vi "Set_Hi-Tec_server.vi"(4 "Client Name":string, 6 "Density Ratio":string, 7 "Strength (% by volume)":dbl min=0.0 max=5.0 format="%.3f", 8 "Stack flowrate (l/min)":dbl format="%.2f", 9 "Mode":enum16{"Control Hi-Tec", "Check Hi-Tec Demands"}(ring)) -> (0 "Flowrates (kg/min)":dbl[](array[numeric]) format="%.2f", 1 "Comment":string)   [LabVIEW 2014]
uses:
  ADAM Client/Sub VIs/ADAM Controls/Ch_description_ADAM.ctl
  ADAM Client/Sub VIs/ADAM Controls/Module_type_ADAM.ctl
  ADAM Client/Sub VIs/ADAM Controls/Function_ADAM.ctl
  ADAM Client/Sub VIs/ADAM Controls/Channel_State.ctl
  ADAM Client/Sub VIs/ADAM Controls/Calib_type_ADAM.ctl
  ADAM Client/Sub VIs/ADAM Controls/Address.ctl
  ADAM Client/Sub VIs/ADAM Controls/Update_scan_value.ctl
  Anemometry/Anemometry Sub Vis/Globals/Gas_management_global.vi
panel:
  # "-Carrier 1 only\n-Carrier 2 only\n-Enter Ratio"
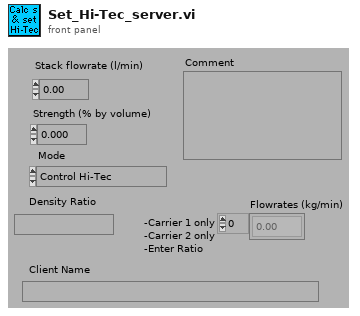
[diagram p1: front panel]
types:
  T1 = enum16{"Append to Global", "Read Global then Clear"}
  T2 = typedef "Calib_type_ADAM.ctl" = enum16{"Raw", "Bx + A", "Cx^2 + Bx + A", "Dx^3 + Cx^2 + Bx + A", "In Band", "Hi-Tec Q", "Hi-Tec M_dot", "Text"}
  T3 = typedef "Module_type_ADAM.ctl" = string
  T4 = typedef "Ch_description_ADAM.ctl" = cluster{"Ch Name":string, "Type":T3, "Function":T5, "Ch State":T6, "Calibration type":T2, "A":dbl, "B":dbl, "C":dbl, "D":dbl, "Comments":string, "Address":T7, "String":string, "Duty":u16}
  T5 = typedef "Function_ADAM.ctl" = enum16{"Analogue Input", "Digital Input", "Event counter", "Event rate", "Analogue Output", "Digital Output", "Relay Output"}
  T6 = typedef "Channel_State.ctl" = enum16{"On", "Off", "Always On", "Always Off"}
  T7 = typedef "Address.ctl" = cluster{"Main":i32, "Ch.":i32, "Sub":i32, "Port Name":string}
  T8 = typedef "Update_scan_value.ctl" = cluster{"Channel Name":string, "New Value":dbl}
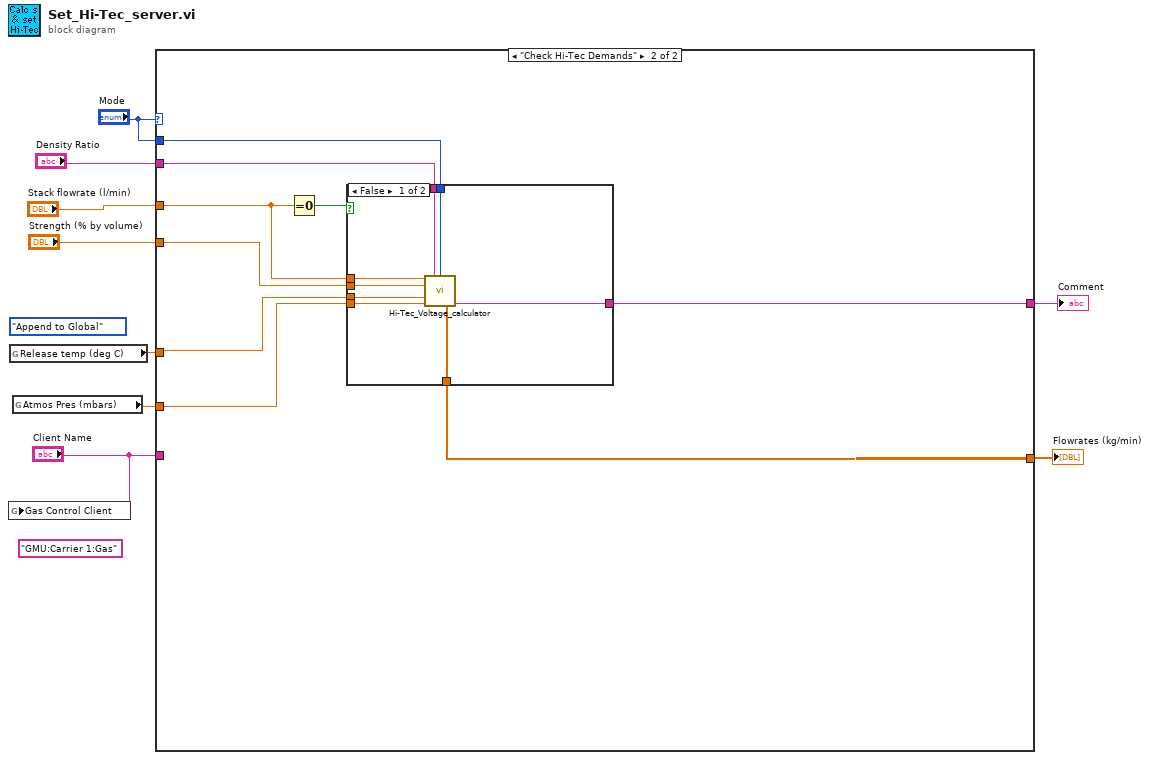
[diagram p0: block diagram]
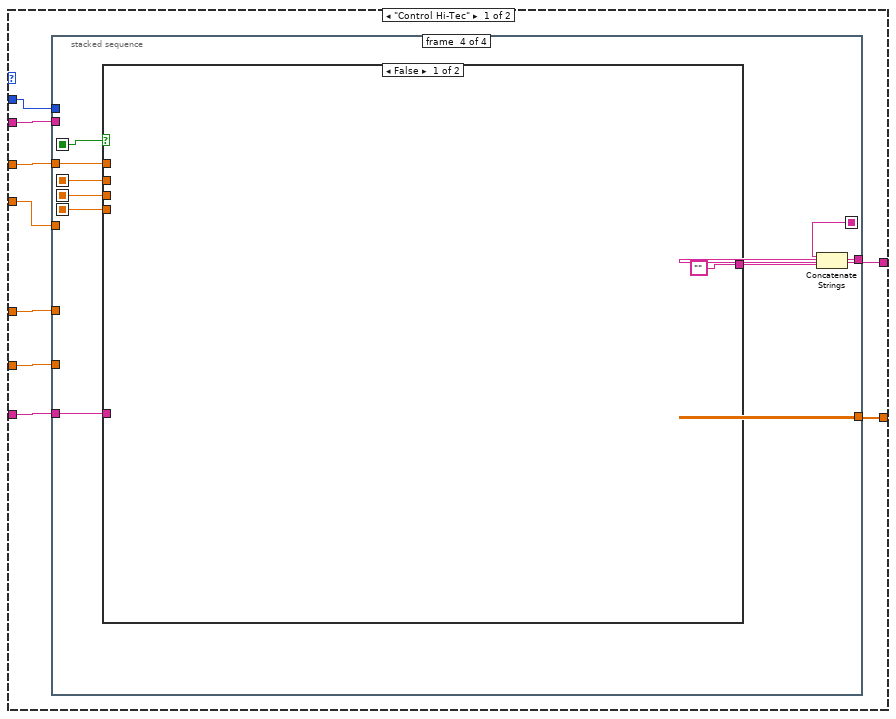
[diagram p2: hidden frame]
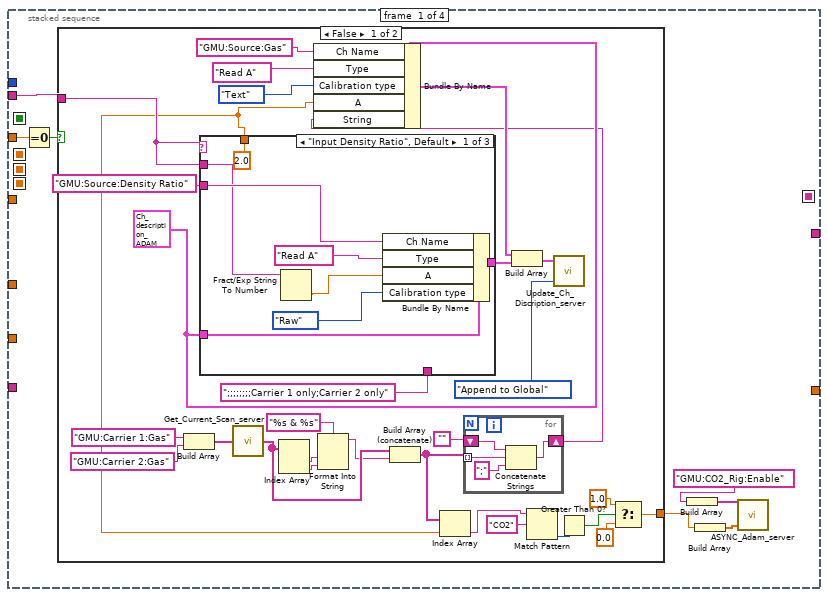
[diagram p3: hidden frame]
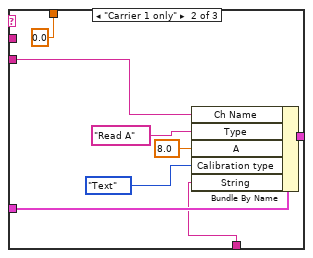
[diagram p4: hidden frame]
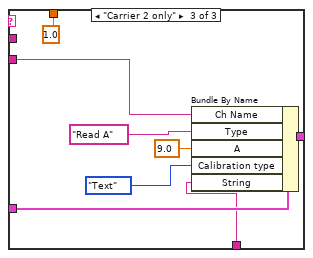
[diagram p5: hidden frame]
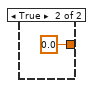
[diagram p6: hidden frame]
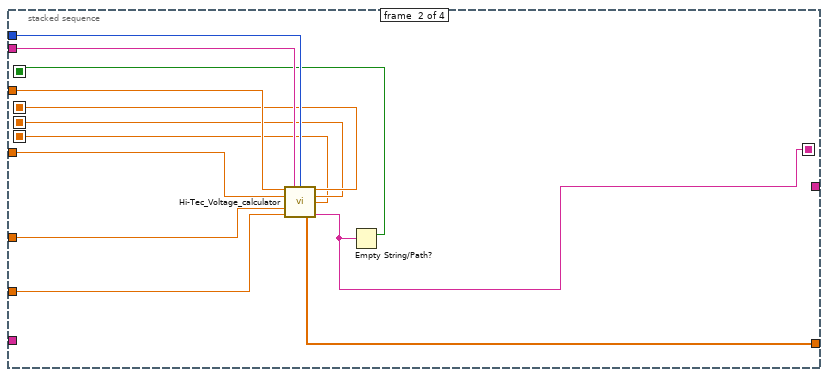
[diagram p7: hidden frame]
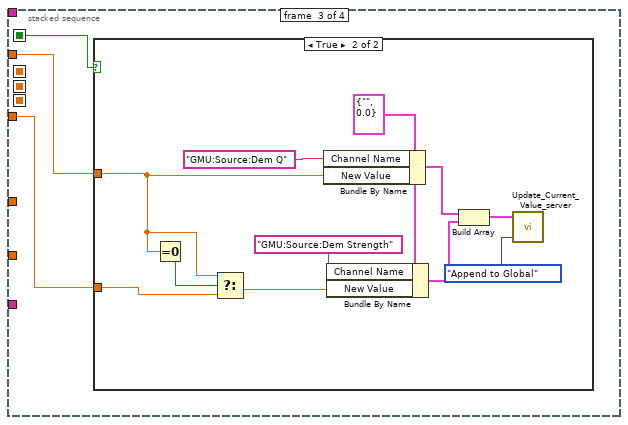
[diagram p8: hidden frame]
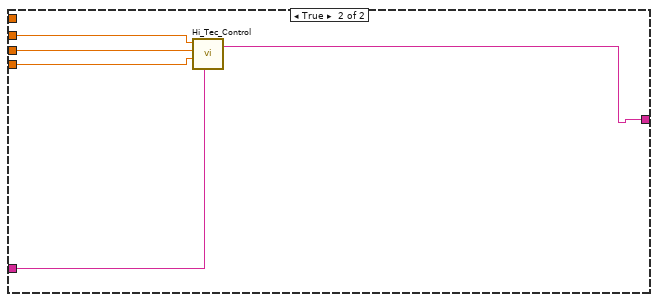
[diagram p10: hidden frame]
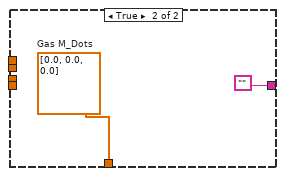
[diagram p11: hidden frame]
diagram:
  (unwired) T1."Append to Global" ("Mode")
  (unwired) "GMU:Carrier 1:Gas"
  n1 = global write "Gas_management_global.vi" "Gas Control Client"("Client Name") -> ()
  n2 = global read "Gas_management_global.vi" "Release temp (deg C)"() -> (w5:dbl)
  n3 = global read "Gas_management_global.vi" "Atmos Pres (mbars)"() -> (w7:dbl)
  n4 = case shown="\"Check Hi-Tec Demands\"" "Mode" {
    tunnel: "Density Ratio" -> [w18 w131]
    tunnel: "Strength (% by volume)" -> [w17 w134]
    tunnel: "Stack flowrate (l/min)" -> [w16 w129]
    tunnel: w5 -> [w15 w133]
    tunnel: w7 -> [w14 w132]
    tunnel: [w13 w130] -> w6
    tunnel: [w12 w127] -> w3
    tunnel: "Mode" -> [w11 w126]
    tunnel: "Client Name" -> [w10 _]
    frame "Control Hi-Tec" {
      n5 = stacked-sequence {
        seq-local: [_ w89 _ _] -> [_ _ w97 w115]
        seq-local: [_ w88 _ _] -> [_ _ _ w119]
        seq-local: [_ w87 _ _] -> [_ _ _ w118]
        seq-local: [_ w86 _ _] -> [_ _ _ w117]
        seq-local: [_ w85 _ _] -> [_ _ _ w112]
        tunnel: w18 -> [w25 w94 _ _]
        tunnel: w17 -> [_ w93 w98 _]
        tunnel: w16 -> [w24 w92 w99 w114]
        tunnel: w15 -> [_ w96 _ _]
        tunnel: w14 -> [_ w95 _ _]
        tunnel: [_ _ _ w113] -> w13
        tunnel: [_ w91 _ _] -> w12
        tunnel: w11 -> [_ w90 _ _]
        tunnel: w10 -> [_ _ _ w116]
        frame #0 {
          n6 = Equal To 0?(x=w24) -> (x = 0?=w23:bool)
          n7 = case shown="False" w23 {
            tunnel: w25 -> [w52 _]
            tunnel: [w26 0.0 ("f")] -> w19
            frame False {
              w43 = T4 {"Ch Name"="", "Type"="", "Function"=enum."Analogue Input", "Ch State"=enum."On", "Calibration type"=enum."Raw", "A"=0.0, "B"=0.0, "C"=0.0, "D"=0.0, "Comments"="", "Address"={"Main"=0, "Ch."=0, "Sub"=0, "Port Name"=""}, "String"="", "Duty"=65535} ("Ch Discription")
              n8 = Build Array("GMU:Carrier 1:Gas", "GMU:Carrier 2:Gas") -> (w51:string[])
              n9 = case shown="\"Input Density Ratio\", Default" w52 {
                tunnel: w43 -> [w67 w75 w83]
                tunnel: "GMU:Source:Density Ratio" -> [w66 w74 w82]
                tunnel: [w63 w70 w78] -> w54
                tunnel: w52 -> [w61 _ _]
                tunnel: ";;;;;;;;Carrier 1 only;Carrier 2 only" -> [_ w69 w77]
                tunnel: [2.0 ("A") 0.0 ("A") 1.0 ("A")] -> w33
                frame "Input Density Ratio", Default {
                  n10 = Fract/Exp String To Number(string=w61) -> (number=w62:dbl)  [unwired: 4 out]
                  n11 = Bundle By Name(cluster=w67, "Ch Name"=w66, "Type"=T3 "Read A", "A"=w62, "Calibration type"=Calib_type_ADAM."Raw") -> (w63:T4)
                }
                frame "Carrier 1 only" {
                  n12 = Bundle By Name(cluster=w75, "Ch Name"=w74, "Type"=T3 "Read A", "A"=8.0 ("Bundle Element"), "Calibration type"=Calib_type_ADAM."Text", "String"=w69) -> (w70:T4)
                }
                frame "Carrier 2 only" {
                  n13 = Bundle By Name(cluster=w83, "Ch Name"=w82, "Type"=T3 "Read A", "A"=9.0 ("Bundle Element"), "Calibration type"=Calib_type_ADAM."Text", "String"=w77) -> (w78:T4)
                }
              }
              n14 = call "Get_Current_Scan_server.vi"("Desired Channels"=w51) -> ("String values"=w39:string[])  [unwired: 2 out]
              n15 = Index Array(array=w39) -> (element #1=w42:string, element #2=w41:string)  [unwired: 2 in]
              n16 = Format Into String(format string="%s & %s", w42, w41) -> (resulting string=w38:string)  [unwired: 2 in, 1 out]
              n17 = Build Array (concatenate)(w39, w38) -> (w34:string[])
              n18 = Index Array(array=w34, index=w33) -> (element=w31:string)
              n19 = for {
                shift-right: [w59] -> w35
                shift-left: "" -> [w58]
                tunnel: w34 -> [w57] mode=indexing
                n20 = Concatenate Strings(w58, w57, ";" ("string")) -> (w59:string)
              }
              n21 = Bundle By Name(cluster=w43, "Ch Name"="GMU:Source:Gas", "Type"=T3 "Read A", "Calibration type"=Calib_type_ADAM."Text", "A"=w33, "String"=w35) -> (w44:T4)
              n22 = Build Array(w44, w54) -> (w53:T4[])
              n23 = Match Pattern(string=w31, regular expression="CO2") -> (offset past match=w30:i32)  [unwired: 1 in, 3 out]
              n24 = call "Update_Ch_Discription_server.vi"("Mode"=T1."Append to Global", "Channels to update In"=w53) -> ()  [unwired: 1 in, 1 out]
              n25 = Greater Than 0?(x=w30) -> (x > 0?=w29:bool)
              n26 = Select(t=1.0, s=w29, f=0.0) -> (s? t:f=w26:dbl)
            }
            frame True {
            }
          }
          n27 = Build Array("GMU:CO2_Rig:Enable") -> (w21:string[])
          n28 = Build Array(w19) -> (w22:dbl[])
          n29 = call "ASYNC_Adam_server.vi"("Values"=w22, "Channel Names"=w21) -> ()  [unwired: 1 in, 3 out]
        }
        frame #1 {
          n30 = call "Hi-Tec_Voltage_calculator.vi"("Stack Flowrate (l/min)"=w92, "Density Ratio"=w94, "Mode"=w90, "Strength (% by volume)"=w93, "Release temp (deg C)"=w96, "Atmos Pres (mbars)"=w95) -> ("Carrier 1 Voltage"=w88:dbl, "Carrier 2 Voltage"=w87:dbl, "Trace Voltage"=w86:dbl, "Flowrates (kg/min)"=w91:dbl[], "Error Comments"=w85:string)  [unwired: 2 in, 3 out]
          n31 = Empty String/Path?(string/path=w85) -> (empty?=w89:bool)
        }
        frame #2 {
          n32 = case shown="True" w97 {
            tunnel: w99 -> [_ w110]
            tunnel: w98 -> [_ w109]
            frame False {
            }
            frame True {
              w104 = T8 {"Channel Name"="", "New Value"=0.0} ("Update Scan Value Cluster")
              n33 = Equal To 0?(x=w110) -> (x = 0?=w101:bool)
              n34 = Select(t=w110, s=w101, f=w109) -> (s? t:f=w100:dbl)
              n35 = Bundle By Name(cluster=w104, "Channel Name"="GMU:Source:Dem Q", "New Value"=w110) -> (w107:T8)
              n36 = Bundle By Name(cluster=w104, "Channel Name"="GMU:Source:Dem Strength", "New Value"=w100) -> (w108:T8)
              n37 = Build Array(w107, w108) -> (w103:T8[])
              n38 = call "Update_Current_Value_server.vi"("Mode"=T1."Append to Global", "Update array in"=w103) -> ()  [unwired: 1 in, 1 out]
            }
          }
        }
        frame #3 {
          n39 = case shown="False" w115 {
            tunnel: w119 -> [_ w125]
            tunnel: w118 -> [_ w124]
            tunnel: w117 -> [_ w123]
            tunnel: w116 -> [_ w122]
            tunnel: w114 -> [_ _]
            tunnel: ["" w121] -> w111
            frame False {
            }
            frame True {
              n40 = call "Hi_Tec_Control.vi"("Carrier 1 Voltage"=w125, "Carrier 2 Voltage"=w124, "Trace Voltage"=w123, "Client Name"=w122) -> ("Scan Comments"=w121:string)  [unwired: 2 out]
            }
          }
          n41 = Concatenate Strings(w112, w111) -> (w113:string)
        }
      }
    }
    frame "Check Hi-Tec Demands" {
      n42 = Equal To 0?(x=w129) -> (x = 0?=w128:bool)
      n43 = case shown="False" w128 {
        tunnel: w134 -> [w142 _]
        tunnel: w133 -> [w141 _]
        tunnel: w132 -> [w140 _]
        tunnel: w131 -> [w139 _]
        tunnel: [w138 ""] -> w130
        tunnel: w129 -> [w137 _]
        tunnel: [w136 w143] -> w127
        tunnel: w126 -> [w135 _]
        frame False {
          n44 = call "Hi-Tec_Voltage_calculator.vi"("Stack Flowrate (l/min)"=w137, "Density Ratio"=w139, "Mode"=w135, "Strength (% by volume)"=w142, "Release temp (deg C)"=w141, "Atmos Pres (mbars)"=w140) -> ("Flowrates (kg/min)"=w136:dbl[], "Error Comments"=w138:string)  [unwired: 1 in, 7 out]
        }
        frame True {
          w143 = dbl[] [0.0, 0.0, 0.0]  # Gas M_Dots
        }
      }
    }
  }
  "Comment" <- w6
  "Flowrates (kg/min)" <- w3
